vi "change tag selection for channel.vi"(5 "channels table":refnum<vi>, 7 "instance identifier":string, 8 "error in":errorcluster, 9 "channels":i32, 10 "Tag":string, 11 "engine configuration in":refnum<class "engine configuration.lvclass">) -> (0 "error out":errorcluster, 3 "engine configuration out":refnum<class "engine configuration.lvclass">)   [LabVIEW 2013, in "Scan Engine editor node.lvclass"]
uses:
  Scan Engine editor node.lvclass
  <vilib>/NI/Module Execution Interface/Engine Configuration/engine configuration.lvclass
  <vilib>/NI/Tag Bus/tag/tag descriptor.lvclass/tag descriptor.ctl
  <vilib>/NI/Tag Bus/tag/write tag name.vi
  <vilib>/NI/Tag Bus Module Framework/channel/TBM channel.lvclass
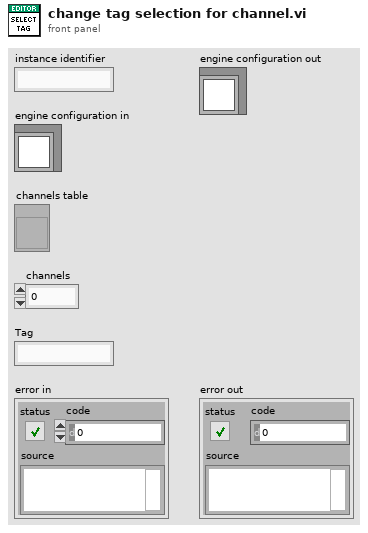
[diagram p1: front panel]
types:
  T1 = typedef "Scan Engine editor node.lvclass/table line.ctl" = cluster{"tag":string, "channel":refnum<class "TBM channel.lvclass">}
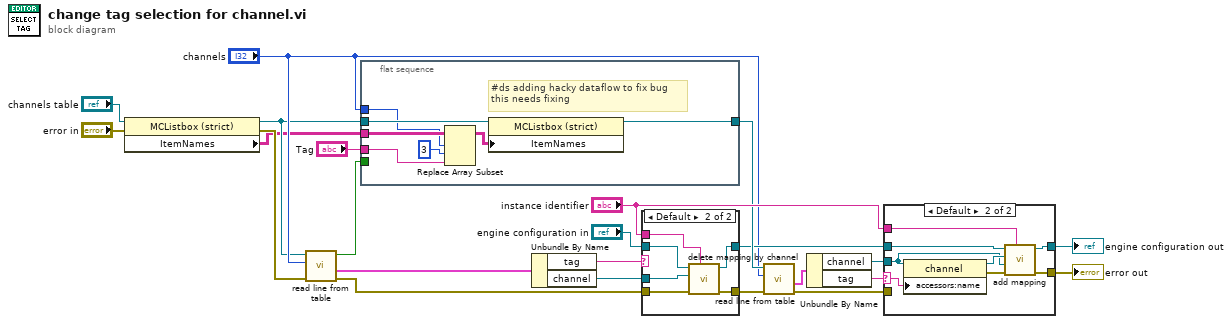
[diagram p0: block diagram]
diagram:
  n1 = property class="MCListbox (strict)"(reference="channels table", error in="error in") -> (reference out=w5:refnum<vi>, error out=w7:errorcluster, "ItemNames"=w4:string[][])
  n2 = call "read line from table.vi"("error in"=w7, "line number"="channels", "operations table"=w5) -> ("error out"=w8:errorcluster, "line"=w11:T1, "empty channel?"=w21:bool)  [unwired: 5 in, 1 out]
  n3 = flat-sequence {
    tunnel: "Tag" -> [w30]
    tunnel: w4 -> [w28]
    tunnel: w5 -> [w26]
    tunnel: "channels" -> [w25]
    tunnel: [w24] -> w16
    tunnel: w21 -> [_]
    frame #0 {
      # "#ds adding hacky dataflow to fix bug\nthis needs fixing"
      n4 = Replace Array Subset(array=w28, new element=w30, index (row)=w25, index (col)=3 ("disabled index (col)")) -> (w29:string[][])
      n5 = property class="MCListbox (strict)"(reference=w26, "ItemNames"=w29) -> (reference out=w24:refnum<vi>)  [unwired: 1 in, 1 out]
    }
  }
  n6 = Unbundle By Name(w11) -> ("tag"=w17:string, "channel"=w18:refnum<class "TBM channel.lvclass">)
  n7 = case shown="Default" w17 {
    tunnel: [w32 w33] -> w19
    tunnel: "instance identifier" -> [_ w34]
    tunnel: w8 -> [w32 w38]
    tunnel: [w31 w37] -> w14
    tunnel: "engine configuration in" -> [w31 w36]
    tunnel: w18 -> [_ w35]
    frame "" {
    }
    frame Default {
      n8 = call <vilib>:"delete mapping by channel.vi"("owner ID"=w34, "error in"=w38, "channel"=w35, "engine configuration in"=w36) -> ("error out"=w33:errorcluster, "engine configuration out"=w37:refnum<class "engine configuration.lvclass">)  [unwired: 6 in]
    }
  }
  n9 = call "read line from table.vi"("error in"=w19, "line number"="channels", "operations table"=w16) -> ("error out"=w9:errorcluster, "line"=w12:T1)  [unwired: 5 in, 2 out]
  n10 = Unbundle By Name(w12) -> ("channel"=w13:refnum<class "TBM channel.lvclass">, "tag"=w15:string)
  n11 = case shown="Default" w15 {
    selector: w15 -> [_ w43]
    tunnel: [w40 w44] -> w10
    tunnel: w9 -> [w40 _]
    tunnel: w13 -> [_ w47]
    tunnel: w14 -> [w39 w45]
    tunnel: [w39 w46] -> w23
    tunnel: "instance identifier" -> [_ w41]
    frame "" {
    }
    frame Default {
      n12 = property class="channel"(reference=w47, "accessors:name"=w43) -> (reference out=w48:refnum<class "TBM channel.lvclass">, error out=w42:errorcluster)  [unwired: 1 in]
      n13 = call <vilib>:"add mapping.vi"("owner ID"=w41, "error in"=w42, "channel"=w47, "tag descriptor"=w48, "engine configuration"=w45) -> ("error out"=w44:errorcluster, "engine configuration out"=w46:refnum<class "engine configuration.lvclass">)  [unwired: 5 in]
    }
  }
  "engine configuration out" <- w23
  "error out" <- w10
